vi "CursorDataGraphMove.vi"(8 "error in (no error)":errorcluster, 9 "ChangeAll":bool, 10 "Data":sgl[][](array[numeric]), 11 "Control-Client in":refnum<class "Control-Client.lvclass">) -> (0 "error out":errorcluster, 1 "Spectra":cluster{"Unités abscisse":dbl[], dbl[]}[](array[cluster]), 2 "Kinetics":cluster{"timedelay":dbl[], dbl[]}[](array[cluster]), 3 "Control-Client out":refnum<class "Control-Client.lvclass">, 4 "Bounds":T2, 6 "Bounds pixels":T1)   [LabVIEW 2018, in "Control-Client.lvclass"]
uses:
  Control-Client.lvclass
  Control-Client.lvclass/Control-Client.ctl
  methods/Read Group #.vi
  Experiments/Experiments_group.lvclass
  Experiments/Experiment.lvclass
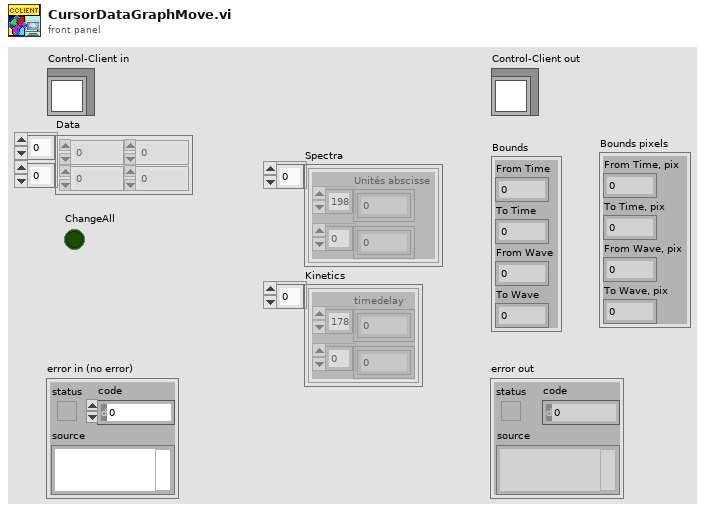
[diagram p1: front panel]
types:
  T1 = cluster{"From Time, pix":i32, "To Time, pix":i32, "From Wave, pix":i32, "To Wave, pix":i32}
  T2 = cluster{"From Time":dbl, "To Time":dbl, "From Wave":dbl, "To Wave":dbl}
  T3 = cluster{"waves slider":refnum<vi>, "times slider":refnum<vi>}
  T4 = cluster{"Max Y pixel":i32, "Min Y pixel":i32, "Max X pixel":i32, "Min X pixel":i32}
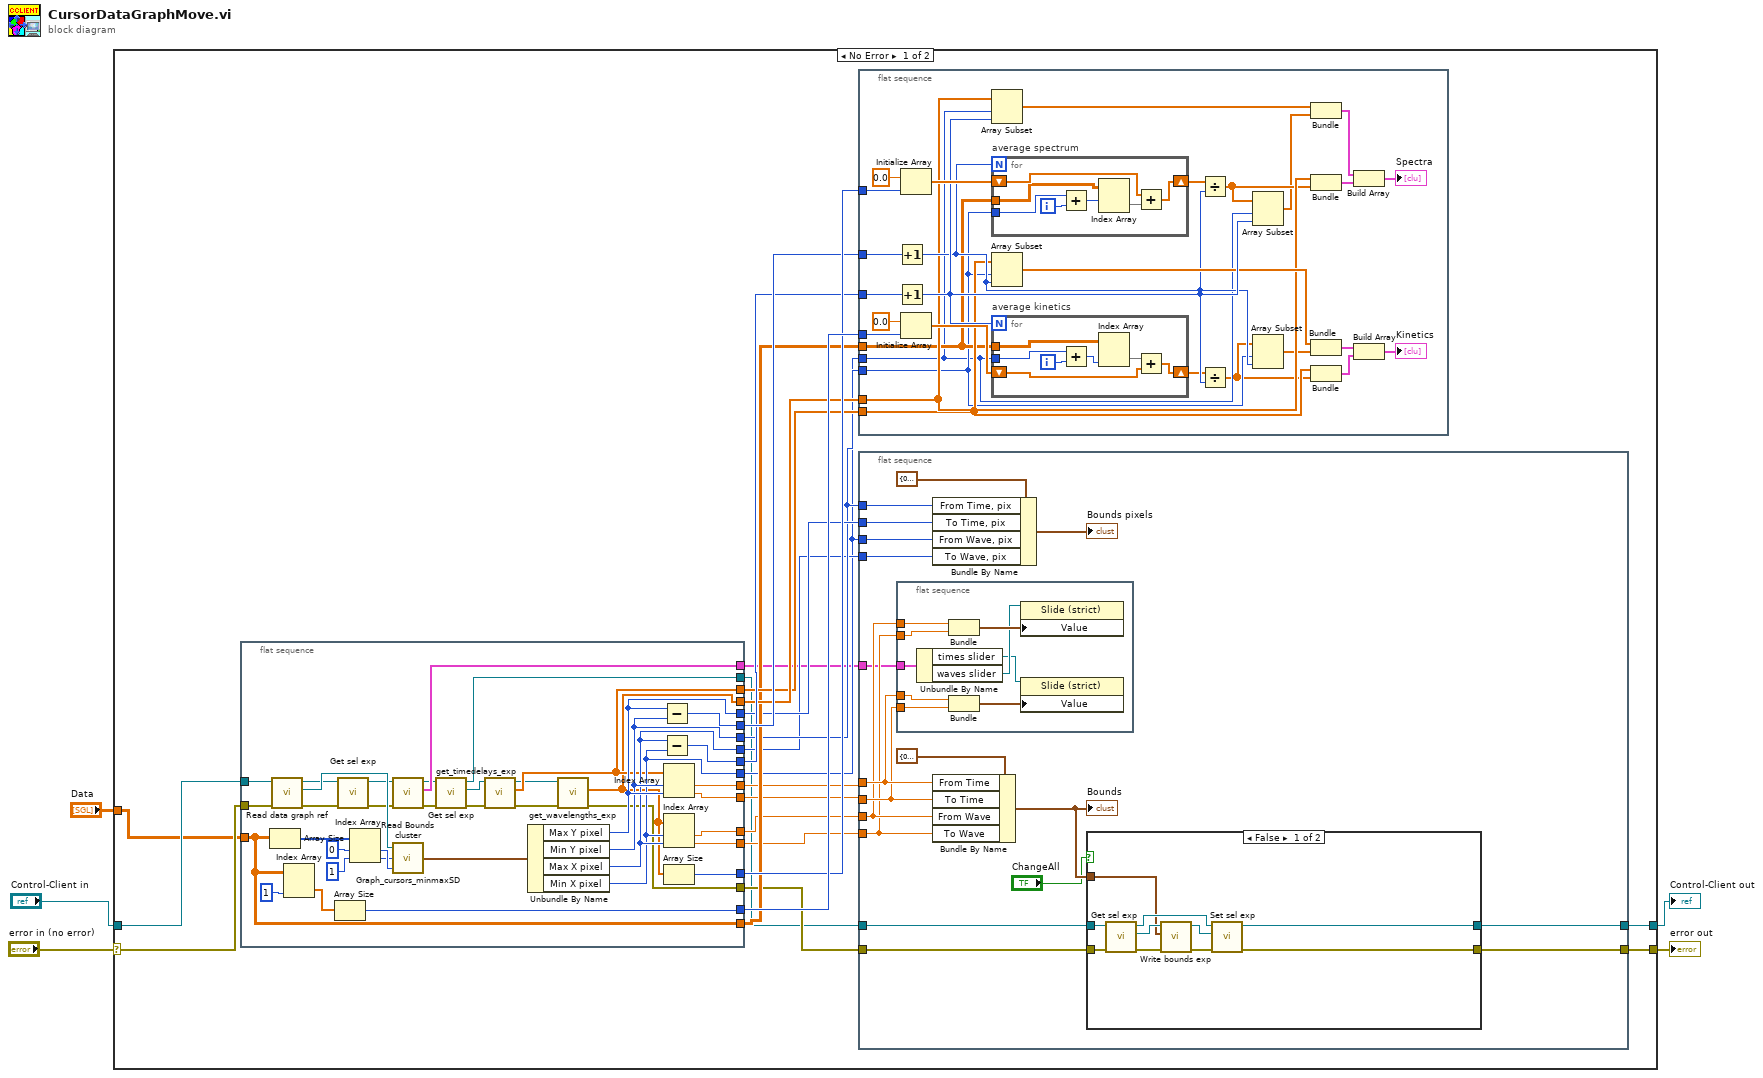
[diagram p0: block diagram]
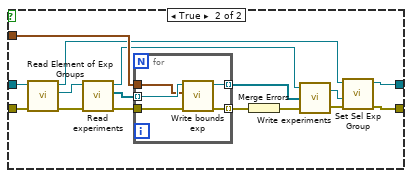
[diagram p2: hidden frame]
diagram:
  n1 = case shown="No Error" "error in (no error)" {
    selector: "error in (no error)" -> [w22 w170]
    tunnel: [w10 w170] -> w4
    tunnel: [w12 w169] -> w2
    tunnel: "Control-Client in" -> [w11 w169]
    tunnel: "Data" -> [w6 _]
    frame No Error {
      n2 = flat-sequence {
        tunnel: [w167] -> w28
        tunnel: [w166] -> w27
        tunnel: [w164] -> w26
        tunnel: [w163] -> w25
        tunnel: [w133] -> w24
        tunnel: [w134] -> w23
        tunnel: w22 -> [w142]
        tunnel: [w140] -> w21
        tunnel: [w161] -> w7
        tunnel: [w160] -> w20
        tunnel: [w159] -> w19
        tunnel: [w158] -> w18
        tunnel: [w157] -> w17
        tunnel: [w156] -> w16
        tunnel: [w155] -> w15
        tunnel: [w154] -> w14
        tunnel: [w153] -> w13
        tunnel: w11 -> [w144]
        tunnel: [w139] -> w9
        tunnel: [w132] -> w8
        tunnel: w6 -> [w140]
        frame #0 {
          n3 = Array Size(array=w140) -> (size(s)=w152:i32[])
          n4 = call "Read data graph ref.vi"("error in (no error)"=w142, "Control-Client in"=w144) -> ("error out"=w143:errorcluster, "Exp data graph ref"=w147:refnum<vi>, "Control-Client out"=w145:refnum<class "Control-Client.lvclass">)  [unwired: 7 in]
          n5 = Index Array(array=w140, index (col)=1 ("disabled index (col)")) -> (element=w168:sgl[])  [unwired: 1 in]
          n6 = Array Size(array=w168) -> (size(s)=w167:i32)
          n7 = call "Get sel exp.vi"("error in (no error)"=w143, "Control-Client in"=w145) -> ("error out"=w141:errorcluster, "Control-Client out"=w146:refnum<class "Control-Client.lvclass">)  [unwired: 7 in, 1 out]
          n8 = Index Array(array=w152, index #1=0 ("index"), index #2=1 ("index")) -> (element #1=w149:i32, element #2=w148:i32)
          n9 = call "Read Bounds cluster.vi"("error in (no error)"=w141, "Control-Client in"=w146) -> ("error out"=w137:errorcluster, "Bounds cluster"=w161:T3, "Control-Client out"=w138:refnum<class "Control-Client.lvclass">)  [unwired: 7 in]
          n10 = call "Graph_cursors_minmaxSD.vi"("Max Y pixel"=w149, "Max X pixel"=w148, "GRAPH EXPERIMENTAL DATA"=w147) -> ("max/min XY pixels"=w165:T4)
          n11 = call "Get sel exp.vi"("error in (no error)"=w137, "Control-Client in"=w138) -> ("error out"=w135:errorcluster, "Sel experiment"=w136:refnum<class "Experiment.lvclass">, "Control-Client out"=w132:refnum<class "Control-Client.lvclass">)  [unwired: 7 in]
          n12 = call "get_timedelays_exp.vi"("error in (no error)"=w135, "Experiment.lvclass in"=w136) -> ("error out"=w131:errorcluster, "timedelays"=w134:dbl[], "Experiment.lvclass out"=w130:refnum<class "Experiment.lvclass">)  [unwired: 7 in]
          n13 = Unbundle By Name(w165) -> ("Max Y pixel"=w156:i32, "Min Y pixel"=w155:i32, "Max X pixel"=w154:i32, "Min X pixel"=w153:i32)
          n14 = call "get_wavelengths_exp.vi"("error in (no error)"=w131, "Experiment.lvclass in"=w130) -> ("error out"=w139:errorcluster, "wavelengths"=w133:dbl[])  [unwired: 7 in, 1 out]
          n15 = Subtract(x=w156, y=w155) -> (x-y=w164:i32)
          n16 = Subtract(x=w154, y=w153) -> (x-y=w163:i32)
          n17 = Index Array(array=w134, index #1=w155, index #2=w156) -> (element #1=w160:dbl, element #2=w159:dbl)
          n18 = Index Array(array=w133, index #1=w153, index #2=w154) -> (element #1=w158:dbl, element #2=w157:dbl)
          n19 = Array Size(array=w133) -> (size(s)=w166:i32)
        }
      }
      n20 = flat-sequence {
        tunnel: w28 -> [w113]
        tunnel: w27 -> [w112]
        tunnel: w26 -> [w107]
        tunnel: w25 -> [w106]
        tunnel: w24 -> [w103]
        tunnel: w23 -> [w102]
        tunnel: w21 -> [w101]
        tunnel: w15 -> [w100]
        tunnel: w13 -> [w99]
        frame #0 {
          n21 = Increment(x=w107) -> (x+1=w104:i32)
          n22 = Increment(x=w106) -> (x+1=w109:i32)
          n23 = Initialize Array(0.0 ("element"), w112) -> (w110:dbl[])
          n24 = Initialize Array(0.0 ("element"), w113) -> (w115:dbl[])
          n25 = Array Subset(array=w103, index=w99, length=w109) -> (w105:dbl[])
          n26 = for "average spectrum" {
            N: w104 -> [_]
            shift-right: [w122] -> w94
            shift-left: w110 -> [w119]
            tunnel: w100 -> [w120]
            tunnel: w101 -> [w118]
            i -> [w121]
            n27 = Add(x=w120, y=w121) -> (x+y=w117:i32)
            n28 = Index Array(array=w118, index (row)=w117) -> (element=w116:sgl[])  [unwired: 1 in]
            n29 = Add(x=w119, y=w116) -> (x+y=w122:dbl[])
          }
          n30 = Array Subset(array=w102, index=w100, length=w104) -> (w108:dbl[])
          n31 = for "average kinetics" {
            N: w109 -> [_]
            tunnel: w101 -> [w129]
            tunnel: w99 -> [w127]
            shift-right: [w123] -> w98
            shift-left: w115 -> [w124]
            i -> [w128]
            n32 = Add(x=w127, y=w128) -> (x+y=w126:i32)
            n33 = Index Array(array=w129, index (col)=w126) -> (element=w125:sgl[])  [unwired: 1 in]
            n34 = Add(x=w125, y=w124) -> (x+y=w123:dbl[])
          }
          n35 = Divide(x=w94, y=w104) -> (x/y=w92:dbl[])
          n36 = Divide(x=w98, y=w109) -> (x/y=w97:dbl[])
          n37 = Array Subset(array=w92, index=w99, length=w109) -> (w91:dbl[])
          n38 = Array Subset(array=w97, index=w100, length=w104) -> (w96:dbl[])
          n39 = Bundle(w105, w91) -> (w90:cluster{dbl[], dbl[]})  [unwired: 1 in]
          n40 = Bundle("wavelengths"=w103, w92) -> (w89:cluster{"wavelengths":dbl[], dbl[]})  [unwired: 1 in]
          n41 = Bundle(w108, w96) -> (w88:cluster{dbl[], dbl[]})  [unwired: 1 in]
          n42 = Bundle("timedelays"=w102, w97) -> (w87:cluster{"timedelays":dbl[], dbl[]})  [unwired: 1 in]
          n43 = Build Array(w90, w89) -> (→"Spectra":cluster{"wavelengths":dbl[], dbl[]}[])
          n44 = Build Array(w88, w87) -> (→"Kinetics":cluster{"timedelays":dbl[], dbl[]}[])
        }
      }
      n45 = flat-sequence {
        tunnel: w20 -> [w46]
        tunnel: w19 -> [w45]
        tunnel: w18 -> [w44]
        tunnel: w17 -> [w43]
        tunnel: w16 -> [w42]
        tunnel: w15 -> [w41]
        tunnel: w14 -> [w40]
        tunnel: w13 -> [w39]
        tunnel: [w38] -> w12
        tunnel: [w37] -> w10
        tunnel: w9 -> [w36]
        tunnel: w8 -> [w35]
        tunnel: w7 -> [w34]
        frame #0 {
          n46 = flat-sequence {
            tunnel: w46 -> [w86]
            tunnel: w45 -> [w85]
            tunnel: w44 -> [w84]
            tunnel: w43 -> [w83]
            tunnel: w34 -> [w82]
            frame #0 {
              n47 = Unbundle By Name(w82) -> ("times slider"=w78:refnum<vi>, "waves slider"=w79:refnum<vi>)
              n48 = Bundle("Numeric"=w84, "Numeric"=w83) -> (w81:cluster{"Numeric":dbl, "Numeric":dbl})  [unwired: 1 in]
              n49 = Bundle("delay"=w86, "delay"=w85) -> (w80:cluster{"delay":dbl, "delay":dbl})  [unwired: 1 in]
              n50 = property class="Slide (strict)"(reference=w79, "Value"=w81) -> ()  [unwired: 1 in, 2 out]
              n51 = property class="Slide (strict)"(reference=w78, "Value"=w80) -> ()  [unwired: 1 in, 2 out]
            }
          }
          n52 = Bundle By Name(cluster=T1 {"From Time, pix"=0, "To Time, pix"=0, "From Wave, pix"=0, "To Wave, pix"=0} ("output cluster"), "From Time, pix"=w41, "To Time, pix"=w42, "From Wave, pix"=w39, "To Wave, pix"=w40) -> (→"Bounds pixels":T1)
          n53 = Bundle By Name(cluster=T2 {"From Time"=0.0, "To Time"=0.0, "From Wave"=0.0, "To Wave"=0.0} ("output cluster"), "From Time"=w46, "To Time"=w45, "From Wave"=w44, "To Wave"=w43) -> (w30:T2)
          "Bounds" <- w30
          n54 = case shown="False" "ChangeAll" {
            tunnel: [w56 w60] -> w38
            tunnel: [w55 w61] -> w37
            tunnel: w36 -> [w54 w71]
            tunnel: w35 -> [w53 w72]
            tunnel: w30 -> [w47 w66]
            frame False {
              n55 = call "Get sel exp.vi"("error in (no error)"=w54, "Control-Client in"=w53) -> ("error out"=w49:errorcluster, "Sel experiment"=w52:refnum<class "Experiment.lvclass">, "Control-Client out"=w50:refnum<class "Control-Client.lvclass">)  [unwired: 7 in]
              n56 = call "Write bounds exp.vi"("error in (no error)"=w49, "Bounds"=w47, "Experiment in"=w52) -> ("error out"=w48:errorcluster, "Experiment out"=w51:refnum<class "Experiment.lvclass">)  [unwired: 7 in]
              n57 = call "Set sel exp.vi"("error in (no error)"=w48, "Experiment"=w51, "Control-Client in"=w50) -> ("error out"=w55:errorcluster, "Control-Client out"=w56:refnum<class "Control-Client.lvclass">)  [unwired: 7 in]
            }
            frame True {
              n58 = call "Read Element of Exp Groups.vi"("error in (no error)"=w71, "Control-Client in"=w72) -> ("error out"=w69:errorcluster, "Experiments_group.lvclass"=w70:refnum<class "Experiments_group.lvclass">, "Control-Client out"=w58:refnum<class "Control-Client.lvclass">)  [unwired: 7 in]
              n59 = call "Read experiments.vi"("error in (no error)"=w69, "Experiments_group.lvclass in"=w70) -> ("error out"=w68:errorcluster, "Experiments"=w67:refnum<class "Experiment.lvclass">[], "Experiments_group.lvclass out"=w65:refnum<class "Experiments_group.lvclass">)  [unwired: 6 in]
              n60 = for {
                tunnel: w68 -> [w73]
                tunnel: w67 -> [w77] mode=indexing
                tunnel: w66 -> [w76]
                tunnel: [w75] -> w64 mode=indexing
                tunnel: [w74] -> w63 mode=indexing
                n61 = call "Write bounds exp.vi"("error in (no error)"=w73, "Bounds"=w76, "Experiment in"=w77) -> ("error out"=w74:errorcluster, "Experiment out"=w75:refnum<class "Experiment.lvclass">)  [unwired: 7 in]
              }
              n62 = Merge Errors(w63) -> (w62:errorcluster)
              n63 = call-dynamic "Write experiments.vi"("error in (no error)"=w62, "Experiments"=w64, "Experiments_group.lvclass in"=w65) -> ("error out"=w57:errorcluster, "Experiments_group.lvclass out"=w59:refnum<class "Experiments_group.lvclass">)
              n64 = call "Set Sel Exp Group.vi"("error in (no error)"=w57, "Exp Group"=w59, "Control-Client in"=w58) -> ("error out"=w61:errorcluster, "Control-Client out"=w60:refnum<class "Control-Client.lvclass">)  [unwired: 7 in]
            }
          }
        }
      }
    }
    frame Error {
    }
  }
  "error out" <- w4
  "Control-Client out" <- w2
